vi "Load node UI optimized.vi"(8 "error in":errorcluster, 10 "node":T12, 11 "state in":T1) -> (0 "error out":errorcluster, 3 "state out":T1)   [LabVIEW 2013]
doc: "This VI will insert the UI from a node into a subpanel."
uses:
  <vilib>/NI/Configuration Framework/Node/NodeRef.ctl
  <vilib>/NI/Configuration Framework/Node/NISE_CEF_Node.lvclass
  Standard Editor/Controls/StateCluster.ctl
  Classes/SystemConfigRepo/SystemConfigRepo.lvclass
  Classes/Systems/Systems.lvclass
  Standard Editor/subVI/SplashScreen/splash screen.ctl
  Standard Editor/subVI/SplashScreen/notifier data.ctl
  <vilib>/NI/Configuration Framework/Node/StandardEvents.ctl
  <vilib>/NI/Configuration Framework/Node/UserEventRef.ctl
  <vilib>/NI/Configuration Framework/Controls/EventCluster.ctl
  <vilib>/NI/Configuration Framework/Node/NodeChangeEvent.ctl
  <vilib>/NI/Configuration Framework/Node/CacheState.ctl
  <vilib>/NI/Configuration Framework/Node/RefreshUIEvent.ctl
  <vilib>/NI/Configuration Framework/Node/StopEvent.ctl
  <vilib>/NI/Configuration Framework/glyph manager/glyph manager.ctl
  <vilib>/picture/picture.llb/imagedata.ctl
  <vilib>/NI/AMC/Message Queue.ctl
  <vilib>/NI/AMC/Message.ctl
  <vilib>/NI/Tools/Keyed Array/KeyedArray.ctl
  <vilib>/NI/Tools/Keyed Array/Tools_KeyedArray.lvlib
  <vilib>/NI/AMC/AMC.lvlib
  <vilib>/NI/Configuration Framework/NISE_CEF_TreeControl.lvlib
  Standard Editor/subVI/SplashScreen/Standard Editor splash screen.lvlib
  <vilib>/NI/Configuration Framework/glyph manager/glyph manager.lvlib
  Standard Editor/Standard Editor.lvlib
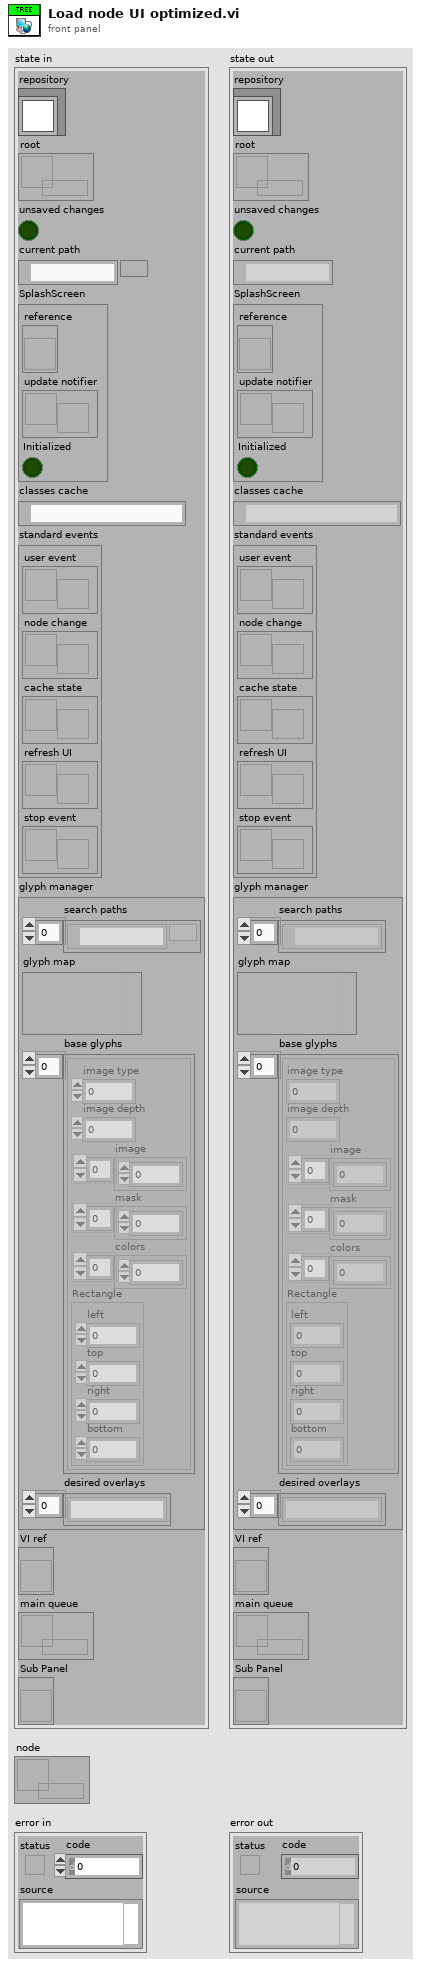
[diagram p1: front panel]
types:
  T1 = typedef "Standard Editor.lvlib/StateCluster.ctl" = cluster{"repository":refnum<class "SystemConfigRepo.lvclass">, "root":refnum<data-value>, "unsaved changes":bool, "current path":path, "SplashScreen":T2, "classes cache":path, "standard events":T3, "glyph manager":T9, "VI ref":refnum<vi>, "main queue":T11, "Sub Panel":refnum<vi>}
  T2 = typedef "Standard Editor splash screen.lvlib/splash screen.ctl" = cluster{"reference":refnum<vi>, "update notifier":refnum<notifier>, "Initialized":bool}
  T3 = typedef "NISE_CEF_Node.lvclass/StandardEvents.ctl" = cluster{"user event":T4, "node change":T5, "cache state":T6, "refresh UI":T7, "stop event":T8}
  T4 = typedef "NISE_CEF_Node.lvclass/UserEventRef.ctl" = refnum<user-event>
  T5 = typedef "NISE_CEF_Node.lvclass/NodeChangeEvent.ctl" = refnum<user-event>
  T6 = typedef "NISE_CEF_Node.lvclass/CacheState.ctl" = refnum<user-event>
  T7 = typedef "NISE_CEF_Node.lvclass/RefreshUIEvent.ctl" = refnum<user-event>
  T8 = typedef "NISE_CEF_Node.lvclass/StopEvent.ctl" = refnum<user-event>
  T9 = typedef "glyph manager.lvlib/glyph manager.ctl" = cluster{"search paths":path[], "glyph map":variant, "base glyphs":T10[], "desired overlays":string[]}
  T10 = typedef "imagedata.ctl" = cluster{"image type":i32, "image depth":i32, "image":u8[], "mask":u8[], "colors":u32[], "Rectangle":cluster{"left":i16, "top":i16, "right":i16, "bottom":i16}}
  T11 = typedef "AMC.lvlib/Message Queue.ctl" = refnum<queue>
  T12 = typedef "NISE_CEF_Node.lvclass/NodeRef.ctl" = refnum<data-value>
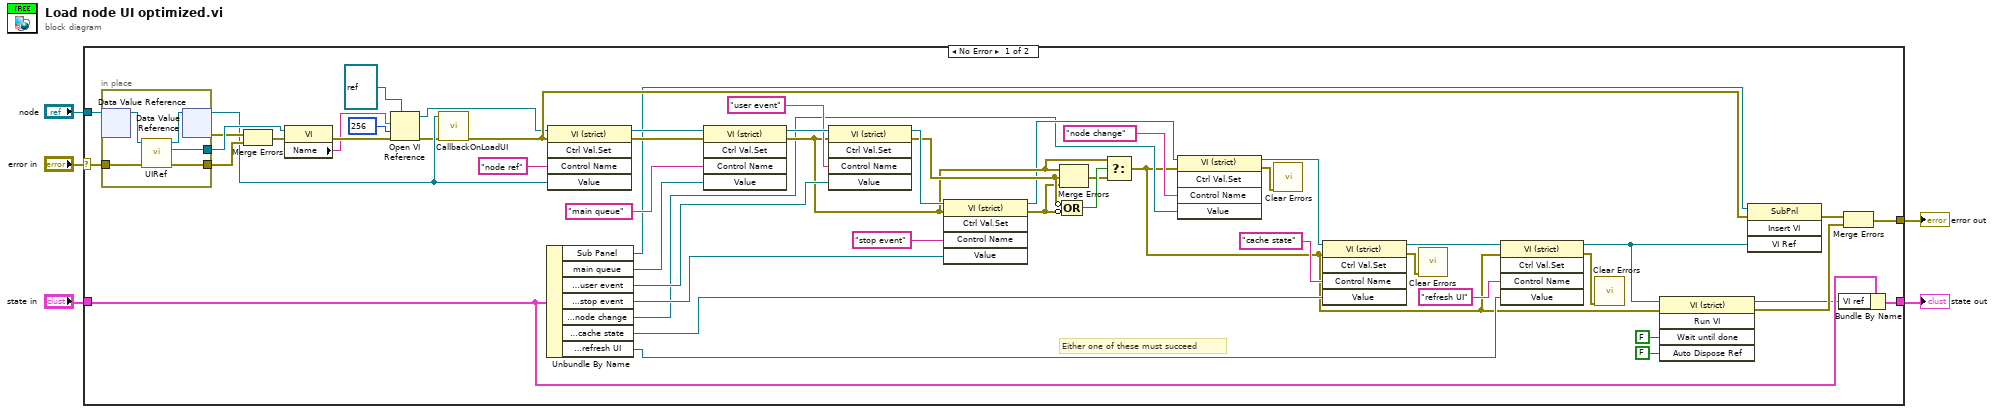
[diagram p0: block diagram]
diagram:
  n1 = case shown="No Error" "error in" {
    selector: "error in" -> [w50 w65]
    tunnel: [w17 w65] -> w4
    tunnel: "node" -> [w48 _]
    tunnel: "state in" -> [w9 w64]
    tunnel: [w8 w64] -> w1
    frame No Error {
      # "Either one of these must succeed"
      n2 = in-place {
        in-place-border: w50 -> [w60]
        in-place-border: [w61] -> w49
        in-place-border: [w59] -> w47
        n3 = in-place-dvr #1(w48) -> (w63:refnum<class "NISE_CEF_Node.lvclass">)  [unwired: 1 out]
        n4 = call-dynamic "UIRef.vi"("error in"=w60, "node in"=w63) -> ("error out"=w59:errorcluster, "VI refnum"=w61:refnum<vi>, "node out"=w62:refnum<class "NISE_CEF_Node.lvclass">)  [unwired: 7 in]
        n5 = in-place-dvr #1(w62) -> (w22:T12, w46:errorcluster)
      }
      n6 = Merge Errors(w46, w47) -> (w45:errorcluster)
      n7 = property class="VI"(reference=w49, error in=w45) -> (error out=w23:errorcluster, "Name"=w14:string)  [unwired: 1 out]
      n8 = Open VI Reference(type specifier VI Refnum (for type only)=refnum<vi> refnum, vi path=w14, options=256, error in (no error)=w23) -> (vi reference=w11:refnum<vi>, error out=w15:errorcluster)  [unwired: 2 in]
      n9 = call <vilib>:"CallbackOnLoadUI.vi"("error in"=w15, "node"=w22) -> ("error out"=w19:errorcluster)  [unwired: 9 in]
      n10 = Unbundle By Name(w9) -> ("Sub Panel"=w6:refnum<vi>, "main queue"=w10:T11, "standard events.user event"=w44:T4, "standard events.stop event"=w42:T8, "standard events.node change"=w29:T5, "standard events.cache state"=w28:T6, "standard events.refresh UI"=w27:T7)
      n11 = invoke class="VI (strict)" method="Ctrl Val.Set"(reference=w11, error in=w19, "Control Name"="node ref", "Value"=w22) -> (reference out=w56:refnum<vi>, error out=w53:errorcluster)  [unwired: 1 in, 3 out]
      n12 = invoke class="VI (strict)" method="Ctrl Val.Set"(reference=w56, error in=w53, "Control Name"="main queue", "Value"=w10) -> (reference out=w52:refnum<vi>, error out=w36:errorcluster)  [unwired: 1 in, 3 out]
      n13 = invoke class="VI (strict)" method="Ctrl Val.Set"(reference=w52, error in=w36, "Control Name"="user event", "Value"=w44) -> (reference out=w43:refnum<vi>, error out=w40:errorcluster)  [unwired: 1 in, 3 out]
      n14 = invoke class="VI (strict)" method="Ctrl Val.Set"(reference=w43, error in=w36, "Control Name"="stop event", "Value"=w42) -> (reference out=w35:refnum<vi>, error out=w39:errorcluster)  [unwired: 1 in, 3 out]
      n15 = Merge Errors(w36, w40, w39) -> (w37:errorcluster)
      n16 = Compound Arithmetic op=OR(invert w40, invert w39) -> (w38:bool)
      n17 = Select(t=w36, s=w38, f=w37) -> (s? t:f=w18:errorcluster)
      n18 = invoke class="VI (strict)" method="Ctrl Val.Set"(reference=w35, error in=w18, "Control Name"="node change", "Value"=w29) -> (reference out=w34:refnum<vi>, error out=w25:errorcluster)  [unwired: 1 in, 3 out]
      n19 = call <vilib>:"Clear Errors.vi"("error in (no error)"=w25) -> ()  [unwired: 6 in, 1 out]
      n20 = invoke class="VI (strict)" method="Ctrl Val.Set"(reference=w34, error in=w18, "Control Name"="cache state", "Value"=w28) -> (reference out=w33:refnum<vi>, error out=w26:errorcluster)  [unwired: 1 in, 3 out]
      n21 = call <vilib>:"Clear Errors.vi"("error in (no error)"=w26) -> ()  [unwired: 6 in, 1 out]
      n22 = invoke class="VI (strict)" method="Ctrl Val.Set"(reference=w33, error in=w18, "Control Name"="refresh UI", "Value"=w27) -> (reference out=w20:refnum<vi>, error out=w24:errorcluster)  [unwired: 1 in, 3 out]
      n23 = call <vilib>:"Clear Errors.vi"("error in (no error)"=w24) -> ()  [unwired: 6 in, 1 out]
      n24 = invoke class="VI (strict)" method="Run VI"(reference=w20, error in=w18, "Wait until done"=FALSE ("Wait Until Done"), "Auto Dispose Ref"=FALSE ("Auto Dispose Reference")) -> (reference out=w7:refnum<vi>, error out=w21:errorcluster)  [unwired: 1 in, 3 out]
      n25 = invoke class="SubPnl" method="Insert VI"(reference=w6, error in=w19, "VI Ref"=w20) -> (error out=w16:errorcluster)  [unwired: 1 in, 3 out]
      n26 = Bundle By Name(cluster=w9, "VI ref"=w7) -> (w8:T1)
      n27 = Merge Errors(w16, w21) -> (w17:errorcluster)
    }
    frame Error {
    }
  }
  "error out" <- w4
  "state out" <- w1
